vi "Example Panel 1.vi"(8 "error in (no error)":errorcluster, 11 "Configuration in":refnum<class "Configuration.lvclass">) -> (0 "error out":errorcluster, 3 "Configuration out":refnum<class "Configuration.lvclass">)   [LabVIEW 2013, in "Example Configuration Dialog.lvlib" / "Example Configuration Dialog.lvclass"]
uses:
  Example Configuration Dialog.lvclass
  Configuration.lvclass
  Example Configuration Dialog.lvclass/Example Configuration Dialog.ctl
panel:
  in  "Paths to Load Measurements From":i32(listbox)
  in  "Delete":bool
  in  "Add":bool
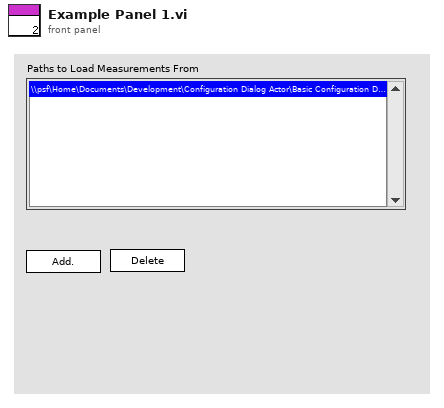
[diagram p1: front panel]
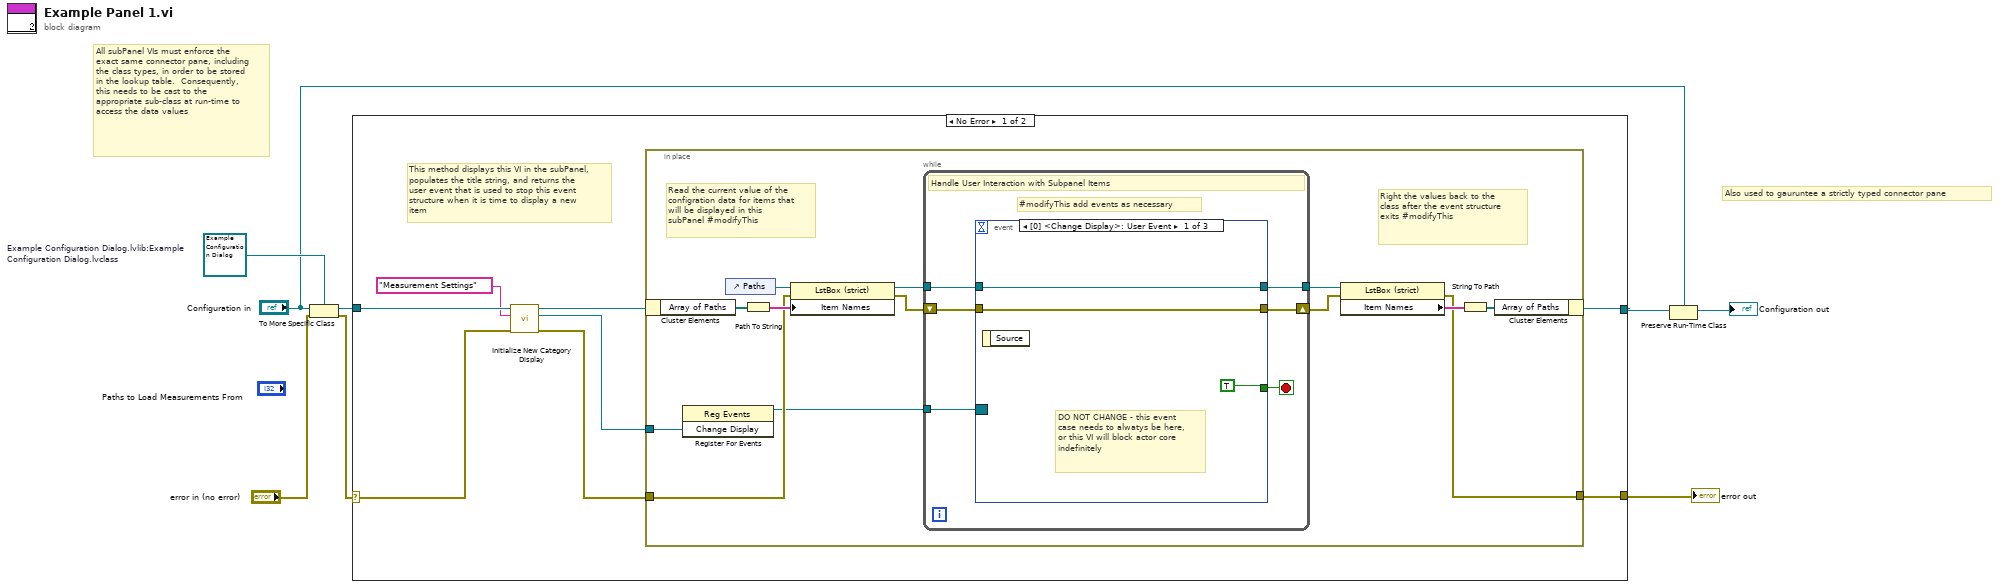
[diagram p0: block diagram]
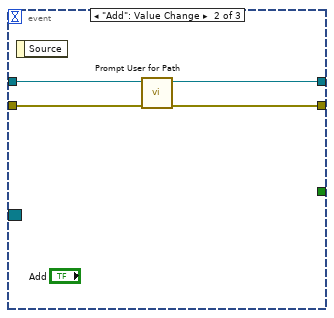
[diagram p2: hidden frame]
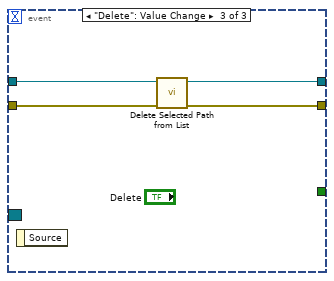
[diagram p3: hidden frame]
diagram:
  w5 = refnum<class "Example Configuration Dialog.lvclass"> refnum  # Example Configuration Dialog.lvlib:Example Configuration Dialog.lvclass
  # "Also used to gauruntee a strictly typed connector pane"
  # "All subPanel VIs must enforce the exact same connector pane, including the class types, in order to be stored in the lookup table.  Consequently, this needs to be cast to the appropriate sub-class at run-time to access the data values"
  n1 = To More Specific Class(target class=w5, reference="Configuration in", error in="error in (no error)") -> (specific class reference=w6:refnum<class "Example Configuration Dialog.lvclass">, error out=w1:errorcluster)
  n2 = case shown="No Error" w1 {
    selector: w1 -> [w10 w47]
    tunnel: w6 -> [w16 w48]
    tunnel: [w14 w48] -> w8
    tunnel: [w12 w47] -> w7
    frame No Error {
      # "This method displays this VI in the subPanel, populates the title string, and returns the user event that is used to stop this event structure when it is time to display a new item"
      n3 = call "Initialize New Category Display.vi"("error in (no error)"=w10, "Name to Display"="Measurement Settings", "Configuration in"=w16) -> ("error out"=w13:errorcluster, "Change Display"=w9:refnum<user-event>, "Configuration Out"=w15:refnum<class "Example Configuration Dialog.lvclass">)  [unwired: 6 in]
      n4 = in-place {
        in-place-border: w13 -> [w27]
        in-place-border: [w24] -> w12
        in-place-border: w9 -> [w23]
        # "Right the values back to the class after the event structure exits #modifyThis"
        # "Read the current value of the configration data for items that will be displayed in this subPanel #modifyThis"
        n5 = in-place-cluster #1(w15) -> ("Array of Paths"=w28:path[])
        n6 = register-events(w23) -> (reference out=w22:refnum<event-registration>)  [unwired: 2 in, 1 out]
        n7 = control-ref of="Paths"() -> (w19:refnum<vi>)
        n8 = Path To String(path=w28) -> (string=w29:string[])
        n9 = property on="Property Node" class="LstBox (strict)"(reference=w19, error in=w27, "Item Names"=w29) -> (reference out=w18:refnum<vi>, error out=w21:errorcluster)
        n10 = while {
          tunnel: w22 -> [w34]
          shift-right: [w33] -> w20
          shift-left: w21 -> [w30]
          tunnel: w18 -> [w32]
          tunnel: [w31] -> w17
          stop <- w35 stop-if-true
          # "#modifyThis add events as necessary"
          # "Handle User Interaction with Subpanel Items"
          n11 = event shown="[0] <Change Display>: User Event" {
            selector: w34 -> [_ _ _]
            dyn-events: _ -> [_ _ _]
            timeout: _ -> [_ _ _]
            tunnel: [TRUE _ _] -> w35
            tunnel: [w36 w40 w44] -> w33
            tunnel: w32 -> [w37 w41 w46]
            tunnel: [w37 w42 w45] -> w31
            tunnel: w30 -> [w36 w39 w43]
            event User Event {
              # "DO NOT CHANGE - this event case needs to alwatys be here, or this VI will block actor core indefinitely"
              n12 = event-data() -> ()  [unwired: 1 in, 1 out]
            }
            event "Add": Value Change {
              n13 = event-data() -> ()  [unwired: 1 in, 1 out]
              n14 = call "Prompt User for Path.vi"("error in (no error)"=w39, "ListBox in"=w41) -> ("error out"=w40:errorcluster, "ListBox out"=w42:refnum<vi>)  [unwired: 8 in]
            }
            event "Delete": Value Change {
              n15 = event-data() -> ()  [unwired: 1 in, 1 out]
              n16 = call "Delete Selected Path from List.vi"("error in (no error)"=w43, "ListBox in"=w46) -> ("error out"=w44:errorcluster, "ListBox out"=w45:refnum<vi>)  [unwired: 8 in]
            }
          }
        }
        n17 = property on="Property Node" class="LstBox (strict)"(reference=w17, error in=w20) -> (error out=w24:errorcluster, "Item Names"=w26:string[])  [unwired: 1 out]
        n18 = String To Path(string=w26) -> (path=w25:path[])
        n19 = in-place-cluster #1("Array of Paths"=w25) -> (w14:refnum<class "Example Configuration Dialog.lvclass">)
      }
    }
    frame Error {
    }
  }
  "error out" <- w7
  n20 = Preserve Run-Time Class(object in=w8, 2:"Configuration in") -> (object out=→"Configuration out":refnum<class "Configuration.lvclass">)  [unwired: 1 in, 1 out]
